vi "RPED Execute.vi"() -> ()   [LabVIEW 2017]
uses:
  RPED Control Type.ctl
  <vilib>/Rock Robotics/WPI/DriverStation/WPI_DriverStationRobotMode2.ctl
  RPED Notifier.ctl
  RPED States.ctl
  RPED Globals.vi
  Utility VIs/Refnum Names.vi
  Robot Global Data.vi
panel:
  out "error out 2":errorcluster
  out "error out":errorcluster
  in  "Time Backward":u32=1500
  in  "Speed Backward":dbl=-0.3
  in  "Speed Forward":dbl=0.7
  in  "Time Forward":u32=500
  in  "Right Back":dbl=-0.2
  in  "Left Back":dbl=-0.2
  in  "Left Forward":dbl=0.6
  in  "Right Forward":dbl=0.6
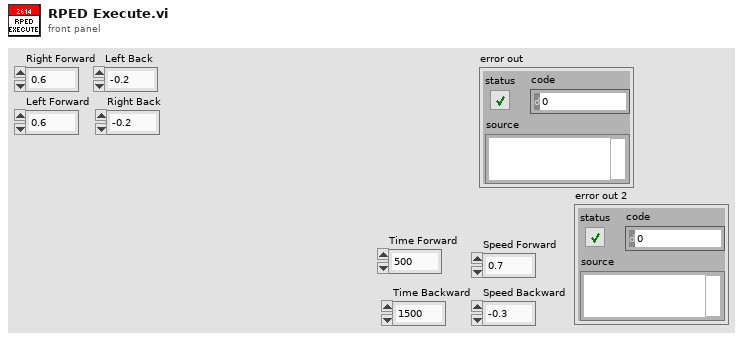
[diagram p1: front panel]
types:
  T1 = typedef "WPI_MotorControlDeviceRef.ctl" = cluster{"DeviceStatus":errorcluster, "Type":T2, "PWM":cluster{"PWM Channel":T3, "DeadBand":T4}, "CAN":cluster{"Device Number":u8, "SetOutput VI Ref":variant, "GetOutput VI Ref":variant, "Enable VI Ref":variant, "Disable VI Ref":variant, "Data":variant}, "Invert":bool, "DIO PWM":cluster{"PWM \"Enable\" Channel":T3, "DIOChannel":T5, "PWM Rate":dbl}}
  T2 = typedef "WPI_MotorControlType.ctl" = enum16{"PWM", "CAN", "DIO PWM"}
  T3 = typedef "FPGA_DIOPWMChannel.ctl" = enum8{"PWM 0", "PWM 1", "PWM 2", "PWM 3", "PWM 4", "PWM 5", "PWM 6", "PWM 7", "PWM 8", "PWM 9", "PWM MXP 0", "PWM MXP 1", "PWM MXP 2", "PWM MXP 3", "PWM MXP 4", "PWM MXP 5", "PWM MXP 6", "PWM MXP 7", "PWM MXP 8", "PWM MXP 9", "Invalid"}
  T4 = typedef "WPI_PWMDeadband.ctl" = cluster{"Name":string, "maxPositivePwm":i32, "minPositivePwm":i32, "centerPwm":i32, "maxNegativePwm":i32, "minNegativePwm":i32, "angularRange":u16}
  T5 = typedef "FPGA_DIOChannel.ctl" = enum8{"DIO 0", "DIO 1", "DIO 2", "DIO 3", "DIO 4", "DIO 5", "DIO 6", "DIO 7", "DIO 8", "DIO 9", "DIO MXP 0", "DIO MXP 1", "DIO MXP 2", "DIO MXP 3", "DIO MXP 4", "DIO MXP 5", "DIO MXP 6", "DIO MXP 7", "DIO MXP 8", "DIO MXP 9", "DIO MXP 10", "DIO MXP 11", "DIO MXP 12", "DIO MXP 13", "DIO MXP 14", "DIO MXP 15", "SPI Port CS1", "SPI Port CS2", "SPI Port CS3", "SPI Port MISO", "SPI Port MOSI", "Invalid"}
  T6 = typedef "RPED Control Type.ctl" = enum16{"No Op", "Left Manual", "Right Manual", "Time", "Left", "Right", "Left_Slow", "Right_Slow", "Left_Distance", "Right_Distance"}
  T7 = typedef "RPED States.ctl" = enum16{"Wait On Button", "Forward", "Backward", "Reset"}
  T8 = typedef "RPED Notifier.ctl" = cluster{"RPED Control Type":T6, "Step":i32, "Left Forward":bool, "Right Forward":bool, "Parameter 1":dbl, "Parameter 2":dbl, "Parameter 3":dbl, "RPED Notifier":refnum<notifier>, "Left Back":bool, "Right Back":bool, "Right":bool, "Left":bool}
  T9 = typedef "WPI_DriverStationRobotMode2.ctl" = enum16{"Autonomous Disabled", "Autonomous Enabled", "Teleop Disabled", "Teleop Enabled", "Disconnected", "Finish", "Test Disabled", "Test Enabled", "Emergency Stopped"}
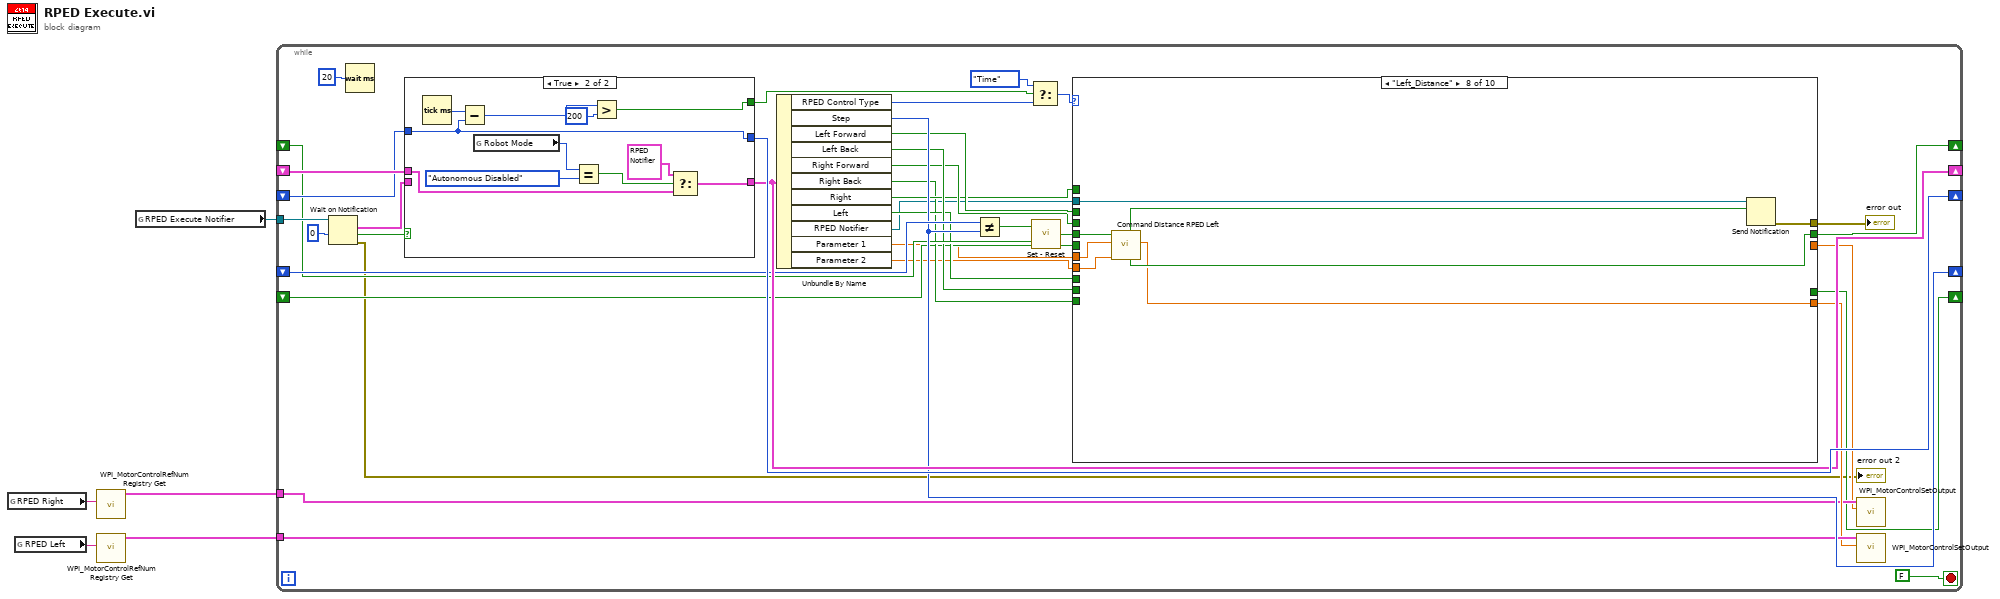
[diagram p0: block diagram]
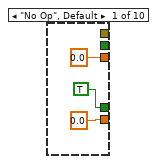
[diagram p2: hidden frame]
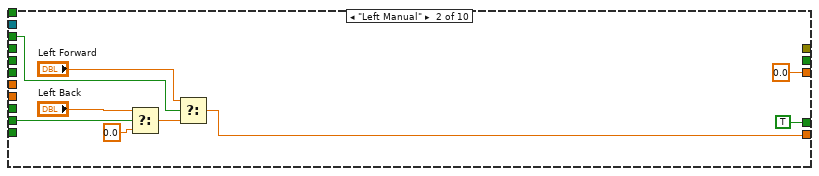
[diagram p3: hidden frame]
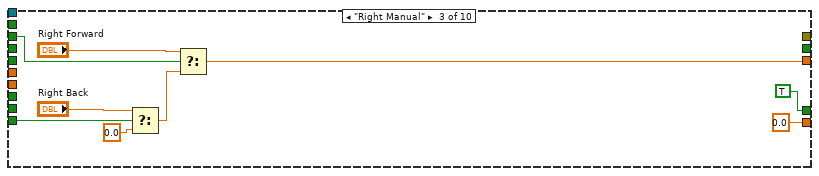
[diagram p4: hidden frame]
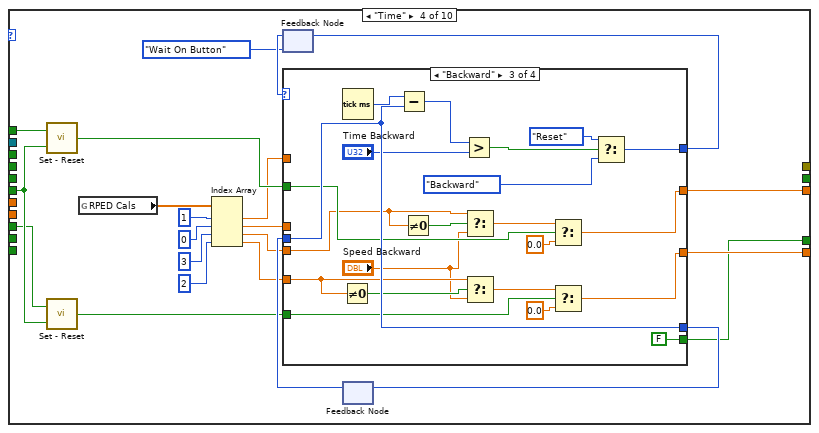
[diagram p5: hidden frame]
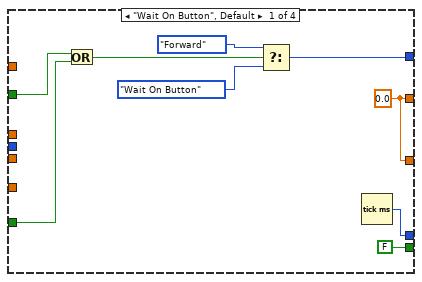
[diagram p6: hidden frame]
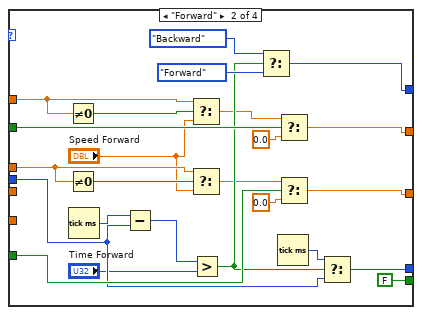
[diagram p7: hidden frame]
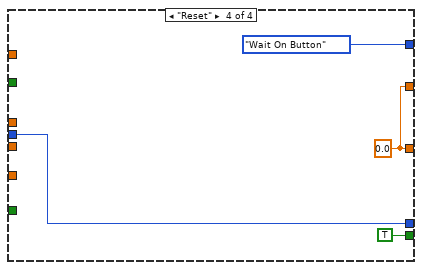
[diagram p8: hidden frame]
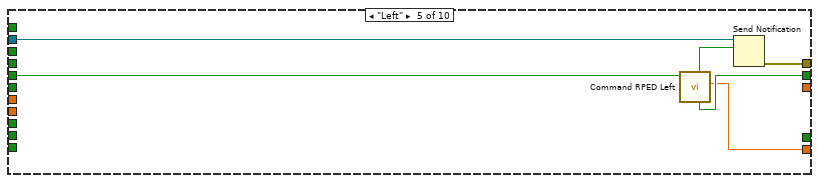
[diagram p9: hidden frame]
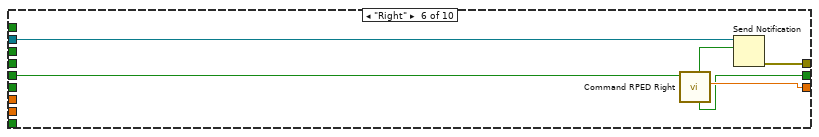
[diagram p10: hidden frame]
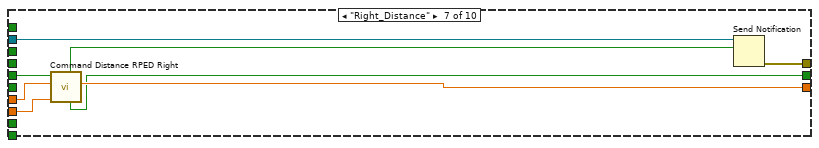
[diagram p11: hidden frame]
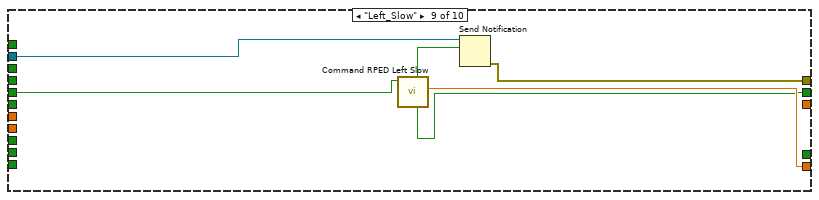
[diagram p12: hidden frame]
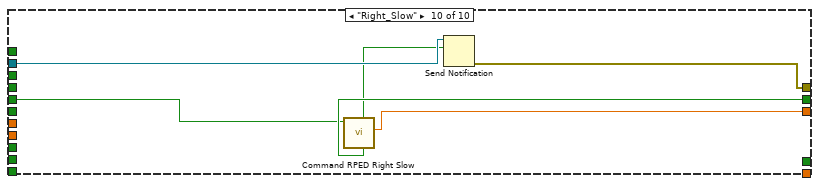
[diagram p13: hidden frame]
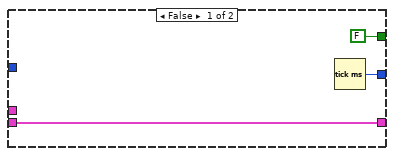
[diagram p14: hidden frame]
diagram:
  n1 = global read "Refnum Names.vi" "RPED Right"() -> (w2:string)
  n2 = global read "Refnum Names.vi" "RPED Left"() -> (w3:string)
  n3 = call <vilib>:"WPI_MotorControlRefNum Registry Get.vi"("refnum name"=w2) -> ("MotorControlDevRef"=w1:T1)  [unwired: 9 in, 1 out]
  n4 = call <vilib>:"WPI_MotorControlRefNum Registry Get.vi"("refnum name"=w3) -> ("MotorControlDevRef"=w4:T1)  [unwired: 9 in, 1 out]
  n5 = global read "RPED Globals.vi" "RPED Execute Notifier"() -> (w5:refnum<notifier>)
  n6 = while {
    tunnel: w5 -> [w40]
    shift-right: [w33] -> _
    shift-left: _ -> [w37]
    shift-right: [w35] -> _
    shift-left: _ -> [w34]
    shift-right: [w28] -> _
    shift-left: _ -> [w29]
    shift-right: [w25] -> _
    shift-left: _ -> [w24]
    tunnel: w4 -> [w22]
    tunnel: w1 -> [w20]
    shift-right: [w12] -> _
    shift-left: _ -> [w11]
    stop <- FALSE stop-if-true
    n7 = Wait on Notification(notifier=w40, timeout in ms (-1)=0) -> (notification=w36:T8, timed out?=w38:bool, error out=→"error out 2":errorcluster)  [unwired: 2 in, 1 out]
    n8 = Wait (ms)(milliseconds to wait=u32 20) -> ()  [unwired: 1 out]
    n9 = case shown="True" w38 {
      tunnel: w37 -> [_ w197]
      tunnel: [w187 w196] -> w33
      tunnel: w36 -> [w187 _]
      tunnel: [w186 w189] -> w35
      tunnel: w34 -> [_ w189]
      tunnel: [FALSE w192] -> w30
      frame False {
        n10 = Tick Count (ms)() -> (millisecond timer value=w186:u32)
      }
      frame True {
        n11 = Tick Count (ms)() -> (millisecond timer value=w195:u32)
        n12 = Subtract(x=w195, y=w189) -> (x-y=w194:u32)
        n13 = global read "Robot Global Data.vi" "Robot Mode"() -> (w191:T9)
        n14 = Equal?(x=w191, y=WPI_DriverStationRobotMode2."Autonomous Disabled") -> (x = y?=w198:bool)
        n15 = Greater?(x=w194, y=u32 200) -> (0:w192:bool)
        n16 = Select(t=T8 {"RPED Control Type"=enum."No Op", "Step"=0, "Left Forward"=FALSE, "Right Forward"=FALSE, "Parameter 1"=0.0, "Parameter 2"=0.0, "Parameter 3"=0.0, "RPED Notifier"=refnum, "Left Back"=FALSE, "Right Back"=FALSE, "Right"=FALSE, "Left"=FALSE} ("RPED Notifier"), s=w198, f=w197) -> (s? t:f=w196:T8)
      }
    }
    n17 = Unbundle By Name(w33) -> ("RPED Control Type"=w32:T6, "Step"=w28:i32, "Left Forward"=w18:bool, "Left Back"=w17:bool, "Right Forward"=w16:bool, "Right Back"=w13:bool, "Right"=w15:bool, "Left"=w14:bool, "RPED Notifier"=w10:refnum<notifier>, "Parameter 1"=w9:dbl, "Parameter 2"=w8:dbl)
    n18 = Not Equal?(x=w29, y=w28) -> (x != y?=w27:bool)
    n19 = Select(t=RPED_Control_Type."Time", s=w30, f=w32) -> (s? t:f=w31:T6)
    n20 = call "Set - Reset.vi"("Reset"=w24, "Set"=w27) -> ("Output"=w26:bool)
    n21 = case shown="\"Left_Distance\"" w31 {
      tunnel: w26 -> [_ _ _ _ w149 w155 w162 w170 w176 w180]
      tunnel: [_ _ _ _ w147 w154 w159 w166 w177 w183] -> w25
      tunnel: [0.0 ("Output") w47 0.0 ("Numeric") w80 w146 _ _ w165 w178 _] -> w21
      tunnel: [0.0 ("Output") 0.0 ("Output") w62 w81 _ w156 w161 _ _ w184] -> w19
      tunnel: w18 -> [_ w52 _ _ _ _ _ _ _ _]
      tunnel: w17 -> [_ w48 _ _ _ _ _ _ _ _]
      tunnel: w16 -> [_ _ w59 _ _ _ _ _ _ _]
      tunnel: w15 -> [_ _ _ w74 _ _ _ _ _ _]
      tunnel: w14 -> [_ _ _ w73 _ _ _ _ _ _]
      tunnel: w13 -> [_ _ w56 _ _ _ _ _ _ _]
      tunnel: [TRUE TRUE TRUE w77 _ _ _ _ _ _] -> w12
      tunnel: w11 -> [_ _ _ w76 _ _ _ _ _ _]
      tunnel: w10 -> [_ _ _ _ w150 w152 w157 w171 w174 w182]
      tunnel: [_ _ _ _ w145 w151 w160 w172 w173 w179] -> w7
      tunnel: w9 -> [_ _ _ _ _ _ w164 w168 _ _]
      tunnel: w8 -> [_ _ _ _ _ _ w163 w167 _ _]
      frame "No Op", Default {
      }
      frame "Left Manual" {
        n22 = Select(t="Left Back", s=w48, f=0.0) -> (s? t:f=w51:dbl)
        n23 = Select(t="Left Forward", s=w52, f=w51) -> (s? t:f=w47:dbl)
      }
      frame "Right Manual" {
        n24 = Select(t="Right Back", s=w56, f=0.0) -> (s? t:f=w61:dbl)
        n25 = Select(t="Right Forward", s=w59, f=w61) -> (s? t:f=w62:dbl)
      }
      frame "Time" {
        n26 = call "Set - Reset.vi"("Reset"=w76, "Set"=w74) -> ("Output"=w79:bool)
        n27 = call "Set - Reset.vi"("Reset"=w76, "Set"=w73) -> ("Output"=w78:bool)
        n28 = global read "RPED Globals.vi" "RPED Cals"() -> (w72:dbl[])
        n29 = Index Array(array=w72, index #1=1 ("index"), index #2=0 ("index"), index #3=3 ("index"), index #4=2 ("index")) -> (element #1=w67:dbl, element #2=w66:dbl, element #3=w65:dbl, element #4=w64:dbl)
        n30 = feedback #1(RPED_States."Wait On Button" ("Enum")) -> (w84:T7)
        n31 = feedback #2() -> (w82:u32)  [unwired: 1 in]
        n32 = case shown="\"Backward\"" w84 {
          tunnel: [w94 w118 w140 RPED_States."Wait On Button" ("Enum")] -> w85
          tunnel: w79 -> [w91 w113 w131 _]
          tunnel: w78 -> [w90 w112 w130 _]
          tunnel: [w88 w104 w137 w141] -> w83
          tunnel: w82 -> [_ w105 w137 w141]
          tunnel: [w87 w114 w132 w144] -> w81
          tunnel: [w87 w111 w129 w144] -> w80
          tunnel: [FALSE FALSE FALSE TRUE] -> w77
          tunnel: w67 -> [_ w100 _ _]
          tunnel: w66 -> [_ w96 _ _]
          tunnel: w65 -> [_ _ w124 _]
          tunnel: w64 -> [_ _ w121 _]
          frame "Wait On Button", Default {
            w87 = 0.0
            n33 = Or(x=w91, y=w90) -> (x .or. y?=w89:bool)
            n34 = Select(t=RPED_States."Forward" ("Enum"), s=w89, f=RPED_States."Wait On Button" ("Enum")) -> (s? t:f=w94:T7)
            n35 = Tick Count (ms)() -> (millisecond timer value=w88:u32)
          }
          frame "Forward" {
            n36 = Not Equal To 0?(x=w100) -> (x != 0?=w101:bool)
            n37 = Not Equal To 0?(x=w96) -> (x != 0?=w97:bool)
            n38 = Tick Count (ms)() -> (millisecond timer value=w108:u32)
            n39 = Subtract(x=w108, y=w105) -> (x-y=w115:u32)
            n40 = Select(t=w100, s=w101, f="Speed Forward") -> (s? t:f=w99:dbl)
            n41 = Select(t=w96, s=w97, f="Speed Forward") -> (s? t:f=w98:dbl)
            n42 = Greater?(x=w115, y="Time Forward") -> (0:w106:bool)
            n43 = Select(t=RPED_States."Backward" ("Enum"), s=w106, f=RPED_States."Forward" ("Enum")) -> (s? t:f=w118:T7)
            n44 = Tick Count (ms)() -> (millisecond timer value=w107:u32)
            n45 = Select(t=w99, s=w113, f=0.0) -> (s? t:f=w114:dbl)
            n46 = Select(t=w98, s=w112, f=0.0) -> (s? t:f=w111:dbl)
            n47 = Select(t=w107, s=w106, f=w105) -> (s? t:f=w104:u32)
          }
          frame "Backward" {
            n48 = Not Equal To 0?(x=w121) -> (x != 0?=w122:bool)
            n49 = Tick Count (ms)() -> (millisecond timer value=w136:u32)
            n50 = Subtract(x=w136, y=w137) -> (x-y=w135:u32)
            n51 = Not Equal To 0?(x=w124) -> (x != 0?=w125:bool)
            n52 = Greater?(x=w135, y="Time Backward") -> (0:w133:bool)
            n53 = Select(t=w124, s=w125, f="Speed Backward") -> (s? t:f=w123:dbl)
            n54 = Select(t=w121, s=w122, f="Speed Backward") -> (s? t:f=w119:dbl)
            n55 = Select(t=w123, s=w131, f=0.0) -> (s? t:f=w132:dbl)
            n56 = Select(t=w119, s=w130, f=0.0) -> (s? t:f=w129:dbl)
            n57 = Select(t=RPED_States."Reset" ("Enum"), s=w133, f=RPED_States."Backward" ("Enum")) -> (s? t:f=w140:T7)
          }
          frame "Reset" {
            w144 = 0.0
          }
        }
        n58 = feedback-in #1(w85) -> ()
        n59 = feedback-in #2(w83) -> ()
      }
      frame "Left" {
        n60 = call "Command RPED Left.vi"("Startup"=w149) -> ("RPED Left"=w146:dbl, "Reinit"=w147:bool, "Completed"=w148:bool)  [unwired: 8 in]
        n61 = Send Notification(notification=w148, notifier=w150) -> (error out=w145:errorcluster)  [unwired: 1 in, 1 out]
      }
      frame "Right" {
        n62 = call "Command RPED Right.vi"("Startup"=w155) -> ("RPED Right"=w156:dbl, "Reinit"=w154:bool, "Completed"=w153:bool)  [unwired: 8 in]
        n63 = Send Notification(notification=w153, notifier=w152) -> (error out=w151:errorcluster)  [unwired: 1 in, 1 out]
      }
      frame "Right_Distance" {
        n64 = call "Command Distance RPED Right.vi"("Timeout"=w163, "Distance"=w164, "Startup"=w162) -> ("RPED Right"=w161:dbl, "Reinit"=w159:bool, "Completed"=w158:bool)  [unwired: 6 in]
        n65 = Send Notification(notification=w158, notifier=w157) -> (error out=w160:errorcluster)  [unwired: 1 in, 1 out]
      }
      frame "Left_Distance" {
        n66 = call "Command Distance RPED Left.vi"("Timeout"=w167, "Distance"=w168, "Startup"=w170) -> ("RPED Left"=w165:dbl, "Reinit"=w166:bool, "Completed"=w169:bool)  [unwired: 6 in]
        n67 = Send Notification(notification=w169, notifier=w171) -> (error out=w172:errorcluster)  [unwired: 1 in, 1 out]
      }
      frame "Left_Slow" {
        n68 = call "Command RPED Left Slow.vi"("Startup"=w176) -> ("RPED Left"=w178:dbl, "Reinit"=w177:bool, "Completed"=w175:bool)  [unwired: 8 in]
        n69 = Send Notification(notification=w175, notifier=w174) -> (error out=w173:errorcluster)  [unwired: 1 in, 1 out]
      }
      frame "Right_Slow" {
        n70 = call "Command RPED Right Slow.vi"("Startup"=w180) -> ("RPED Right"=w184:dbl, "Reinit"=w183:bool, "Completed"=w181:bool)  [unwired: 8 in]
        n71 = Send Notification(notification=w181, notifier=w182) -> (error out=w179:errorcluster)  [unwired: 1 in, 1 out]
      }
    }
    "error out" <- w7
    n72 = call <vilib>:"WPI_MotorControlSetOutput.vi"("Output"=w19, "MotorControlDevRef"=w20) -> ()  [unwired: 7 in, 3 out]
    n73 = call <vilib>:"WPI_MotorControlSetOutput.vi"("Output"=w21, "MotorControlDevRef"=w22) -> ()  [unwired: 7 in, 3 out]
  }
